vi "Change to Background Color.vi"(7 "change type":T1, 11 "item names":string[](array[string])) -> (3 "background colors":u32[](array[colorbox]))   [LabVIEW 2020, in "AIM MIL-STD-1553 System Explorer.lvlib" / "Implementation.lvlib" / "Refresh.lvlib"]
uses:
  Refresh.lvlib
  Change Type.ctl
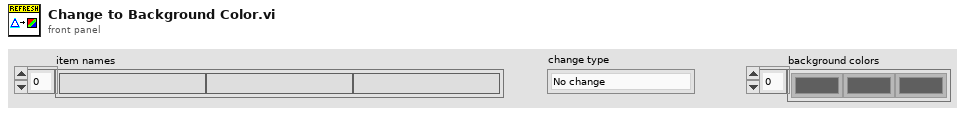
[diagram p1: front panel]
types:
  T1 = typedef "AIM MIL-STD-1553 System Explorer.lvlib/Implementation.lvlib/Refresh.lvlib/Change Type.ctl" = enum16{"No change", "Modify", "Add", "Remove"}
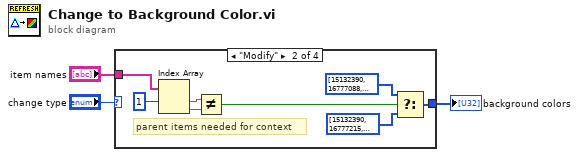
[diagram p0: block diagram]
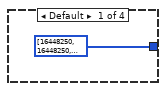
[diagram p2: hidden frame]
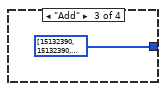
[diagram p3: hidden frame]
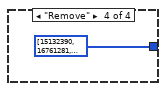
[diagram p4: hidden frame]
diagram:
  n1 = case shown="\"Modify\"" "change type" {
    tunnel: [u32[] [16448250, 16448250, 16448250] ("Bulk Cells:Background Colors") w11 u32[] [15132390, 15132390, 11468718] ("Bulk Cells:Background Colors") u32[] [15132390, 16761281, 15132390] ("Bulk Cells:Background Colors")] -> w1
    tunnel: "item names" -> [_ w7 _ _]
    frame Default {
    }
    frame "Modify" {
      # "parent items needed for context"
      n2 = Index Array(array=w7, index #1=1 ("index")) -> (element #1=w9:string, element #2=w8:string)  [unwired: 1 in]
      n3 = Not Equal?(x=w9, y=w8) -> (x != y?=w5:bool)
      n4 = Select(t=u32[] [15132390, 16777088, 16777088] ("Bulk Cells:Background Colors"), s=w5, f=u32[] [15132390, 16777215, 16777215] ("Bulk Cells:Background Colors")) -> (s? t:f=w11:u32[])
    }
    frame "Add" {
    }
    frame "Remove" {
    }
  }
  "background colors" <- w1
